vi "test timing reporting enable disable.vi"() -> ()   [LabVIEW 2013, in "std eng tests.lvlib"]
uses:
  std eng tests.lvlib
  Configuration/Standard Engine Configuration.lvclass
  Configuration/timing reporting tags.ctl
panel:
  out "set partial ok":bool
  out "empty":errorcluster
  out "normal":errorcluster
  out "overwrite unset":errorcluster
  out "overwrite":errorcluster
  out "partial":errorcluster
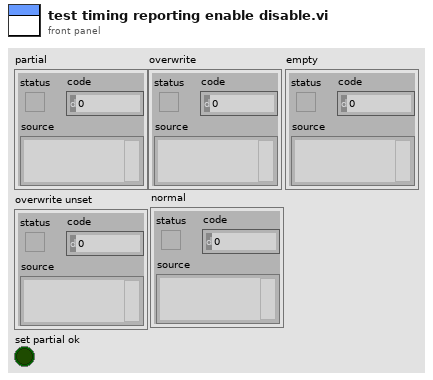
[diagram p1: front panel]
types:
  T1 = typedef "Standard Engine Configuration.lvclass/timing reporting tags.ctl" = cluster{"late index (bool)":string, "late count index (U32)":string, "current dt ns(U64)":string}
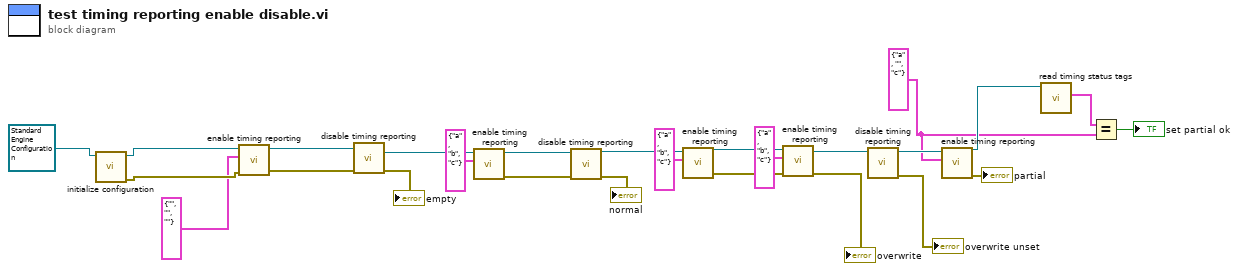
[diagram p0: block diagram]
diagram:
  w2 = T1 {"late index (bool)"="a", "late count index (U32)"="", "current dt ns(U64)"="c"} ("timing reporting")
  n1 = call-dynamic "initialize configuration.vi"("configuration in"=refnum<class "Standard Engine Configuration.lvclass"> refnum ("Standard Engine Configuration")) -> ("error out"=w24:errorcluster, "configuration out"=w25:refnum<class "Standard Engine Configuration.lvclass">)  [unwired: 8 in, 1 out]
  n2 = call "enable timing reporting.vi"("error in"=w24, "timing reporting"=T1 {"late index (bool)"="", "late count index (U32)"="", "current dt ns(U64)"=""}, "Standard Engine Configuration in"=w25) -> ("error out"=w22:errorcluster, "Standard Engine Configuration out"=w23:refnum<class "Standard Engine Configuration.lvclass">)  [unwired: 7 in]
  n3 = call "disable timing reporting.vi"("error in"=w22, "Standard Engine Configuration in"=w23) -> ("error out"=→"empty":errorcluster, "Standard Engine Configuration out"=w20:refnum<class "Standard Engine Configuration.lvclass">)  [unwired: 8 in]
  n4 = call "enable timing reporting.vi"("timing reporting"=T1 {"late index (bool)"="a", "late count index (U32)"="b", "current dt ns(U64)"="c"}, "Standard Engine Configuration in"=w20) -> ("error out"=w18:errorcluster, "Standard Engine Configuration out"=w19:refnum<class "Standard Engine Configuration.lvclass">)  [unwired: 8 in]
  n5 = call "disable timing reporting.vi"("error in"=w18, "Standard Engine Configuration in"=w19) -> ("error out"=→"normal":errorcluster, "Standard Engine Configuration out"=w17:refnum<class "Standard Engine Configuration.lvclass">)  [unwired: 8 in]
  n6 = call "enable timing reporting.vi"("timing reporting"=T1 {"late index (bool)"="a", "late count index (U32)"="b", "current dt ns(U64)"="c"}, "Standard Engine Configuration in"=w17) -> ("error out"=w15:errorcluster, "Standard Engine Configuration out"=w16:refnum<class "Standard Engine Configuration.lvclass">)  [unwired: 8 in]
  n7 = call "enable timing reporting.vi"("error in"=w15, "timing reporting"=T1 {"late index (bool)"="a", "late count index (U32)"="b", "current dt ns(U64)"="c"}, "Standard Engine Configuration in"=w16) -> ("error out"=→"overwrite":errorcluster, "Standard Engine Configuration out"=w14:refnum<class "Standard Engine Configuration.lvclass">)  [unwired: 7 in]
  n8 = call "disable timing reporting.vi"("Standard Engine Configuration in"=w14) -> ("error out"=→"overwrite unset":errorcluster, "Standard Engine Configuration out"=w13:refnum<class "Standard Engine Configuration.lvclass">)  [unwired: 9 in]
  n9 = call "enable timing reporting.vi"("timing reporting"=w2, "Standard Engine Configuration in"=w13) -> ("error out"=→"partial":errorcluster, "Standard Engine Configuration out"=w4:refnum<class "Standard Engine Configuration.lvclass">)  [unwired: 8 in]
  n10 = call "read timing status tags.vi"("Standard Engine Configuration in"=w4) -> ("timing reporting"=w3:T1)  [unwired: 8 in, 2 out]
  n11 = Equal?(x=w3, y=w2) -> (x = y?=→"set partial ok":bool)
